vi "Read Payload.vi"(8 "error in":errorcluster, 11 "CutomOOB_Tx in":refnum<class "CIFCustomOOB_Tx.lvclass">) -> (0 "error out":errorcluster, 2 "data":T1, 3 "CutomOOB_Tx out":refnum<class "CIFCustomOOB_Tx.lvclass">)   [LabVIEW 2021, in "CIFCustomOOB_Tx.lvclass"]
uses:
  CIFCustomOOB_Tx.lvclass
  CIFCustomOOB_Tx.lvclass/CIFCustomOOB_Tx.ctl
  CIFUtilities/CIFOutOfBand/CIFOutOfBand.lvclass
  Typedef/Payload.ctl
  D:/dev/CIF-LVCore/src/CIFUtilities/CIFOutOfBand/CIFOutOfBand.lvclass
  D:/dev/CIF-LVCore/src/CIFTemplatePlugin/OOB/OOB_Tx/CIFCustomOOB_Tx.lvclass
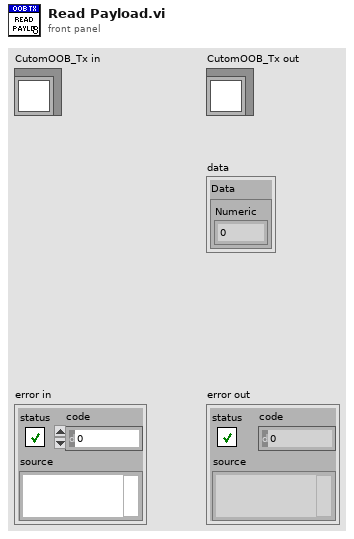
[diagram p1: front panel]
types:
  T1 = typedef "CIFCustomOOB_Tx.lvclass/Payload.ctl" = cluster{"Data":cluster{"Numeric":i32}}
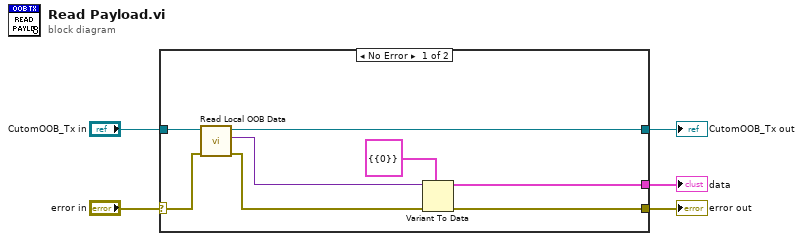
[diagram p0: block diagram]
diagram:
  n1 = case shown="No Error" "error in" {
    selector: "error in" -> [w12 w15]
    tunnel: [w11 w15] -> w5
    tunnel: [w7 w14] -> w4
    tunnel: "CutomOOB_Tx in" -> [w13 w14]
    tunnel: [w6 _] -> w1
    frame No Error {
      n2 = call "Read Local OOB Data.vi"("error in"=w12, "OOB in"=w13) -> ("error out"=w10:errorcluster, "Local OOB Data"=w9:variant, "OOB in"=w7:refnum<class "CIFCustomOOB_Tx.lvclass">)  [unwired: 7 in]
      n3 = Variant To Data(error in=w10, type=T1 {"Data"={"Numeric"=0}}, Variant=w9) -> (data=w6:T1, error out=w11:errorcluster)
    }
    frame Error {
    }
  }
  "error out" <- w5
  "CutomOOB_Tx out" <- w4
  "data" <- w1
